vi "ReadTexttoArray02.vi"(4 "delimiter (Tab)":string="\t", 5 "index":i32=1, 6 "transpose (no:F)":bool, 7 "format (%.3f)":string="%.3f", 8 "max characters/row  (no limit:0)":i32, 9 "start of read offset (chars.:0)":i32, 10 "number of rows (all:-1)":i32=-1, 11 "file path (dialog if empty)":path=path "C:/Users/Academia Sinica/Desktop/AutoSampler _GB/AutoSampler.txt") -> (0 "EOF?":bool, 1 "mark after read (chars.)":i32=13, 2 "number":i32=20, 3 "all rows":string[][](array[string])=[["20"], ["20"], ["20"], ["0"]])   [LabVIEW 2018]
doc: "Reads a specified number of lines or rows from a numeric text file beginning at a specified character offset and converts the data to a 2D, single-precision array of numbers."
panel:
  out "size(s)":i32=4
  in  "type (empty)":string[][](array[string])
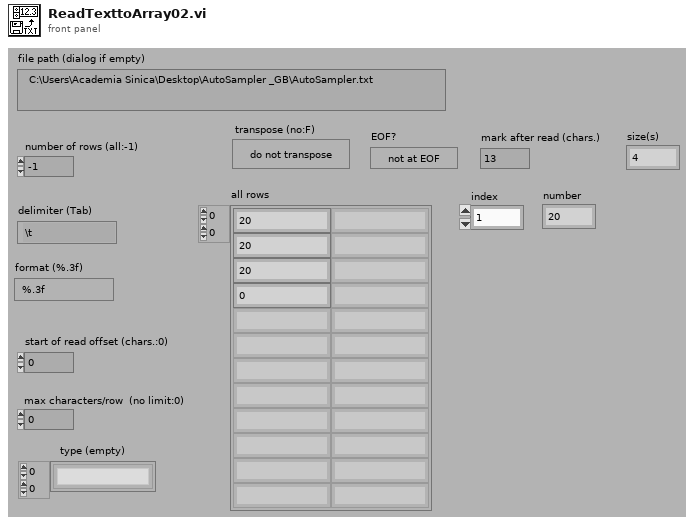
[diagram p1: front panel]
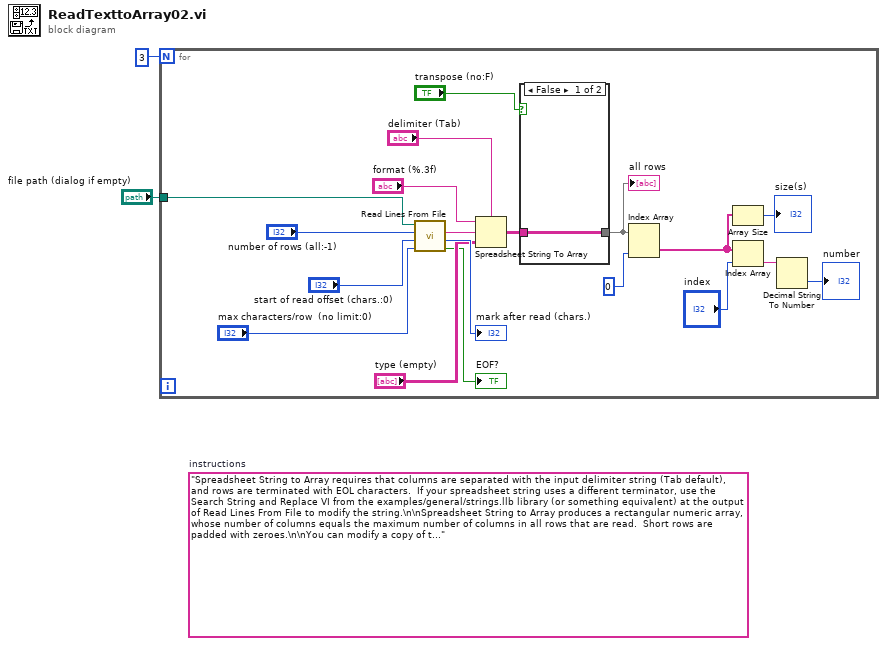
[diagram p0: block diagram]
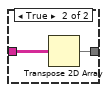
[diagram p2: hidden frame]
diagram:
  (unwired) "Spreadsheet String to Array requires that columns are separated with the input delimiter string (Tab default), and rows are terminated with EOL characters.  If your spreadsheet string uses a different terminator, use the Search String and Replace VI from the examples/general/strings.llb library (or something equivalent) at the output of Read Lines From File to modify the string.\n\nSpreadsheet String to Array produces a rectangular numeric array, whose number of columns equals the maximum number of columns in all rows that are read.  Short rows are padded with zeroes.\n\nYou can modify a copy of this VI to return the file contents into arrays of strings by changing all rows, first row, and type (empty) arrays to string arrays and by setting the format to %s."  # instructions
  n1 = for {
    N: 3 -> [_]
    tunnel: "file path (dialog if empty)" -> [w3]
    n2 = call <vilib>:"Read Lines From File.vi"("file path (dialog if empty)"=w3, "number of lines (all:-1)"="number of rows (all:-1)", "start of read offset (chars.:0)"="start of read offset (chars.:0)", "[max characters per line]  (no limit:0)"="max characters/row  (no limit:0)") -> ("line string"=w18:string, "mark after read (chars.)"=→"mark after read (chars.)":i32, "EOF?"=→"EOF?":bool)  [unwired: 2 in, 1 out]
    n3 = Spreadsheet String To Array(delimiter (Tab)="delimiter (Tab)", format string="format (%.3f)", spreadsheet string=w18, array type (2D Dbl)="type (empty)") -> (array=w16:string[][])
    n4 = case shown="False" "transpose (no:F)" {
      tunnel: [w22 w24] -> w10
      tunnel: w16 -> [w22 w23]
      frame False {
      }
      frame True {
        n5 = Transpose 2D Array(2D array=w23) -> (transposed array=w24:string[][])
      }
    }
    "all rows" <- w10
    n6 = Index Array "Index Array"(array=w10, index (col)=0) -> (element=w8:string[])  [unwired: 1 in]
    n7 = Array Size(array=w8) -> (size(s)=→"size(s)":i32)
    n8 = Index Array(array=w8, index="index") -> (element=w6:string)
    n9 = Decimal String To Number(string=w6) -> (number=→"number":i32)  [unwired: 2 in, 1 out]
  }
